vi "Server Log Panel.vi"(8 "error in":errorcluster, 11 "open window (false)":variant) -> (0 "error out":errorcluster, 3 "text ref":variant)   [LabVIEW 2020]
doc: "This panel shows log of server traffic."
uses:
  other/GUI Panel Control Action.ctl
  varilib/SGUI Assign References Mode.ctl
  varilib/varilib.lvlib
panel:
  in  "btn clear":bool
  in  "btn log exit":bool
  out "str log":string caption="Log"
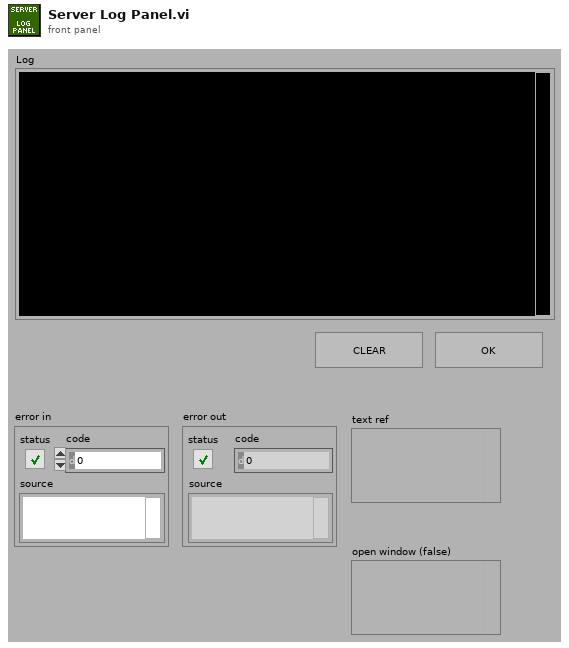
[diagram p1: front panel]
types:
  T1 = typedef "varilib.lvlib/SGUI Assign References Mode.ctl" = enum16{"Add to stack", "Overwrite", "Release last", "Release ID"}
  T2 = typedef "GUI Panel Control Action.ctl" = enum16{"Open panel", "Close panel", "Bring To Front"}
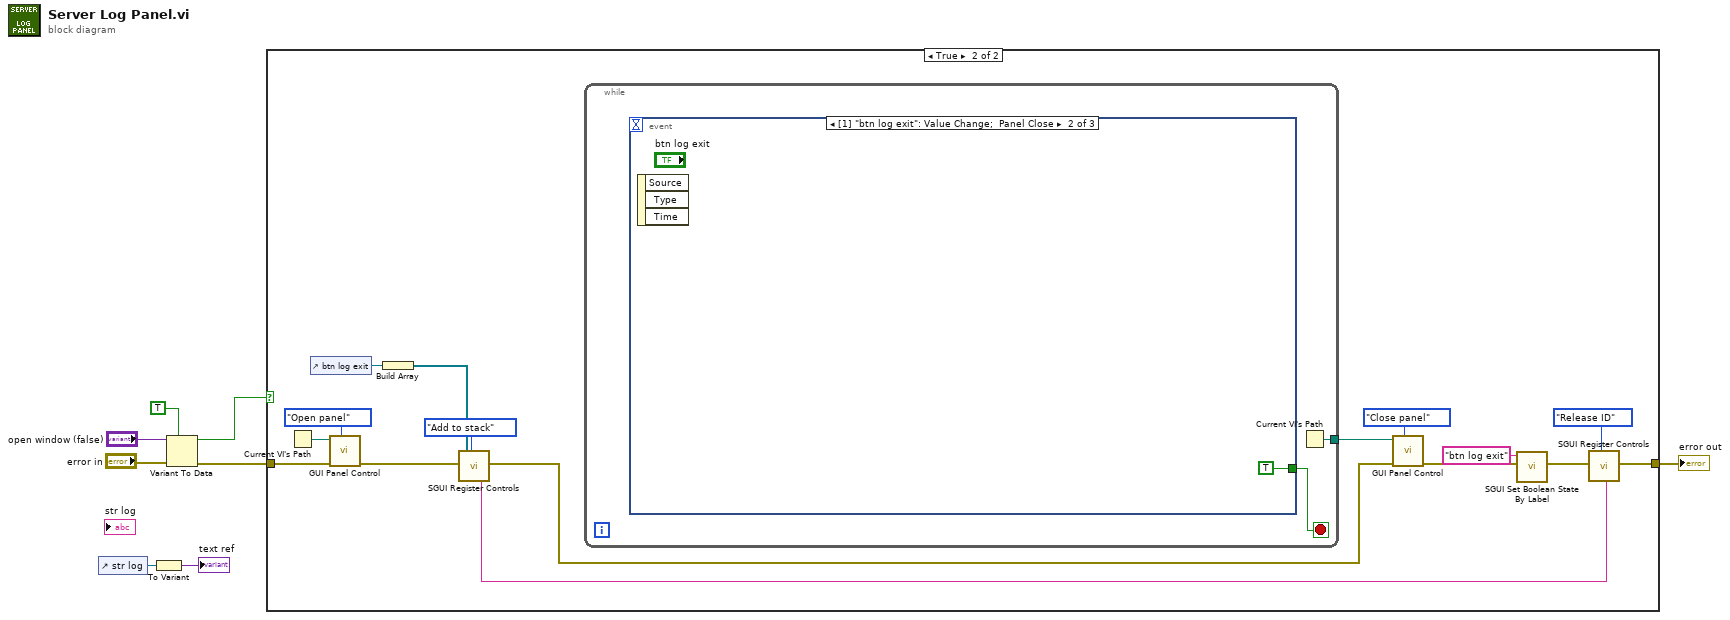
[diagram p0: block diagram]
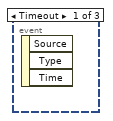
[diagram p3: hidden frame]
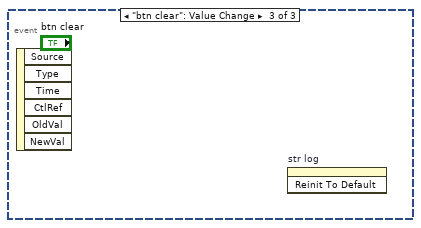
[diagram p4: hidden frame]
diagram:
  n1 = control-ref of="str log"() -> (w7:refnum<vi>)
  n2 = To Variant(anything=w7) -> (Variant=→"text ref":variant)
  n3 = Variant To Data(error in="error in", type=TRUE, Variant="open window (false)") -> (data=w1:bool, error out=w2:errorcluster)
  n4 = case shown="True" w1 {
    tunnel: w2 -> [w9 w25]
    tunnel: [w9 w15] -> w8
    frame False {
    }
    frame True {
      n5 = Current VI's Path() -> (path=w22:path)
      n6 = control-ref of="btn log exit"() -> (w19:refnum<vi>)
      n7 = call "GUI Panel Control.vi"("action (open panel)"=GUI_Panel_Control_Action."Open panel", "error in (no error)"=w25, "vi path"=w22) -> ("error out"=w17:errorcluster)  [unwired: 8 in]
      n8 = Build Array(w19) -> (w18:refnum<vi>[])
      n9 = call "SGUI Register Controls.vi"("error in"=w17, "control references (empty)"=w18, "register mode (overwrite)"=SGUI_Assign_References_Mode."Add to stack") -> ("assigned ID"=w13:string, "error out"=w16:errorcluster)  [unwired: 14 in, 1 out]
      n10 = while {
        tunnel: [w26] -> w21
        stop <- w27 stop-if-true
        n11 = event shown="[1] \"btn log exit\": Value Change;  Panel Close" {
          selector: _ -> [_ _ _]
          dyn-events: _ -> [_ _ _]
          timeout: _ -> [_ _ _]
          tunnel: [_ TRUE _] -> w27
          event Timeout {
            n12 = event-data() -> ()  [unwired: 1 in, 3 out]
          }
          event "btn log exit": Value Change; Panel Close {
            n13 = event-data() -> ()  [unwired: 1 in, 3 out]
          }
          event "btn clear": Value Change {
            n14 = event-data() -> ()  [unwired: 1 in, 6 out]
            n15 = invoke on="str log" class="Str" method="Reinit To Default"() -> ()  [unwired: 3 in, 3 out]
          }
        }
        n16 = Current VI's Path() -> (path=w26:path)
      }
      n17 = call "GUI Panel Control.vi"("action (open panel)"=GUI_Panel_Control_Action."Close panel", "error in (no error)"=w16, "vi path"=w21) -> ("error out"=w12:errorcluster)  [unwired: 8 in]
      n18 = call "SGUI Set Boolean State By Label.vi"("error in"=w12, "control label(s) ('btn stop')"="btn log exit") -> ("error out"=w11:errorcluster)  [unwired: 8 in, 1 out]
      n19 = call "SGUI Register Controls.vi"("error in"=w11, "register mode (overwrite)"=SGUI_Assign_References_Mode."Release ID", "controls ID (empty)"=w13) -> ("error out"=w15:errorcluster)  [unwired: 14 in, 2 out]
    }
  }
  "error out" <- w8
